vi "SetPathInfo.vi"(0 "reference":refnum<class "StateDiagramGraph.lvclass">, 1 "StateDiagramData.VI-Path":path, 2 "StateDiagramData.ShowOption":T1, 5 "error in (no error)":errorcluster) -> (14 "reference out":refnum<class "StateDiagramGraph.lvclass">, 15 "NodesBounds":T2 {"height" format="%.2f"; "width" format="%.2f"; "y" format="%.2f"; "x" format="%.2f"}, 19 "error out":errorcluster)   [LabVIEW 2014, in "StateDiagramGraph.lvclass"]
doc: "draw"
uses:
  <resource>/Framework/Providers/Open_GDS/UML/StateDiagramGraph_class/StateDiagramGraph.lvclass
  <resource>/Framework/Providers/Open_GDS/UML/General/Rectangle/Rectangle Rectangle2D.ctl
  <resource>/Framework/Providers/Open_GDS/UML/StateDiagramGraph_class/private/ViPathShowOption.ctl
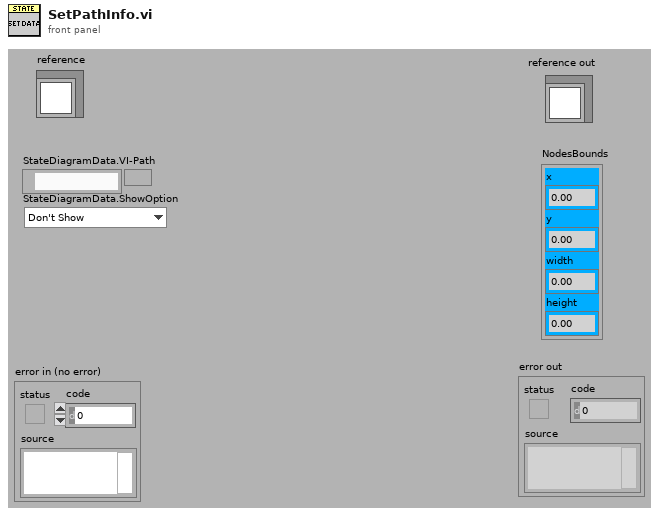
[diagram p1: front panel]
types:
  T1 = typedef "StateDiagramGraph.lvclass/ViPathShowOption.ctl" = enum16{"Don't Show", "Show Relative Path", "Show Absolute Path"}
  T2 = typedef "Rectangle Rectangle2D.ctl" = cluster{"x":dbl, "y":dbl, "width":dbl, "height":dbl}
  T3 = typedef "StateDiagramGraph.lvclass/ObjectAttributes.ctl" = cluster{"StateDiagramData":T4}
  T4 = typedef "StateDiagramGraph.lvclass/StateDiagramData.ctl" = cluster{"VI-Path":path, "ShowOption":T1}
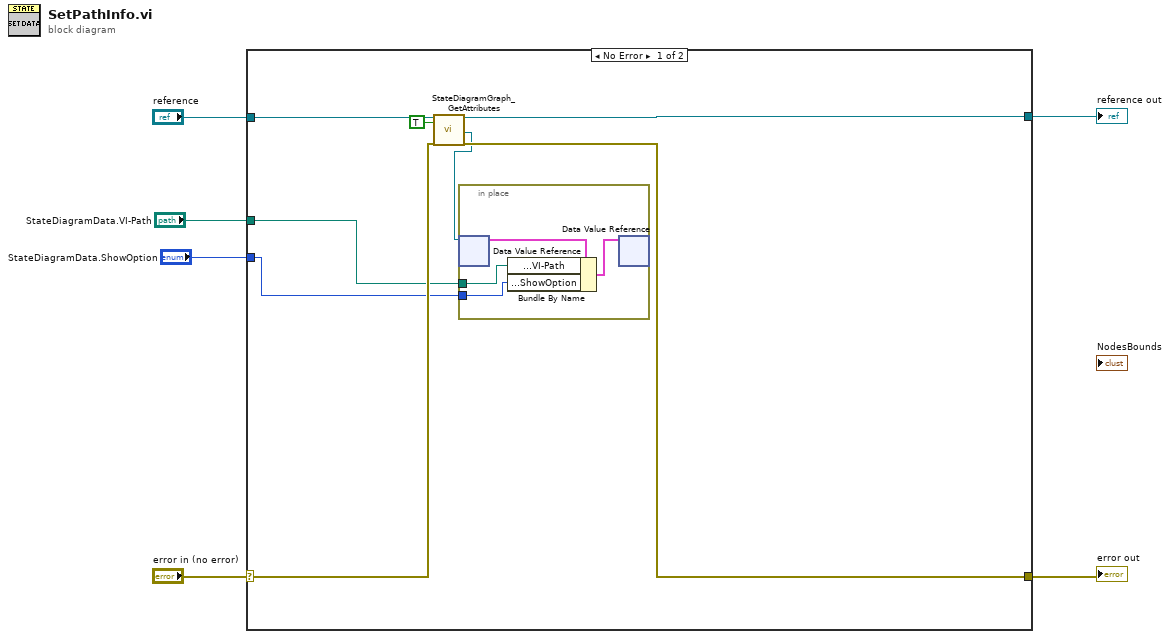
[diagram p0: block diagram]
diagram:
  n1 = case shown="No Error" "error in (no error)" {
    selector: "error in (no error)" -> [w11 w19]
    tunnel: "reference" -> [w14 w20]
    tunnel: [w12 w19] -> w4
    tunnel: [w13 w20] -> w3
    tunnel: "StateDiagramData.VI-Path" -> [w8 _]
    tunnel: "StateDiagramData.ShowOption" -> [w7 _]
    frame No Error {
      n2 = call <resource>:"StateDiagramGraph_GetAttributes.vi"("reference in"=w14, "OnlyGetDvrReference(False)"=TRUE, "error in (no error)"=w11) -> ("reference out"=w13:refnum<class "StateDiagramGraph.lvclass">, "DataRef"=w9:refnum<data-value>, "error out"=w12:errorcluster)  [unwired: 13 in, 1 out]
      n3 = in-place {
        in-place-border: w8 -> [w17]
        in-place-border: w7 -> [w16]
        n4 = in-place-dvr #1(w9) -> (w18:T3)  [unwired: 1 out]
        n5 = Bundle By Name(cluster=w18, "StateDiagramData.VI-Path"=w17, "StateDiagramData.ShowOption"=w16) -> (w15:T3)
        n6 = in-place-dvr #1(w15) -> ()  [unwired: 2 out]
      }
    }
    frame Error {
    }
  }
  "reference out" <- w3
  "error out" <- w4
